vi "Delete Device Record.vi"(8 "error in (no error)":errorcluster, 10 "Device":string, 11 "Configuration in":refnum<class "Configuration.lvclass">) -> (0 "error out":errorcluster, 3 "Configuration out":refnum<class "Configuration.lvclass">)   [LabVIEW 2023, in "Configuration.lvlib" / "Configuration.lvclass"]
uses:
  Library/Configuration.lvclass
  Library/Configuration.lvclass/Configuration.ctl
  <vilib>/Utility/config.llb/NI_LVConfig.lvlib
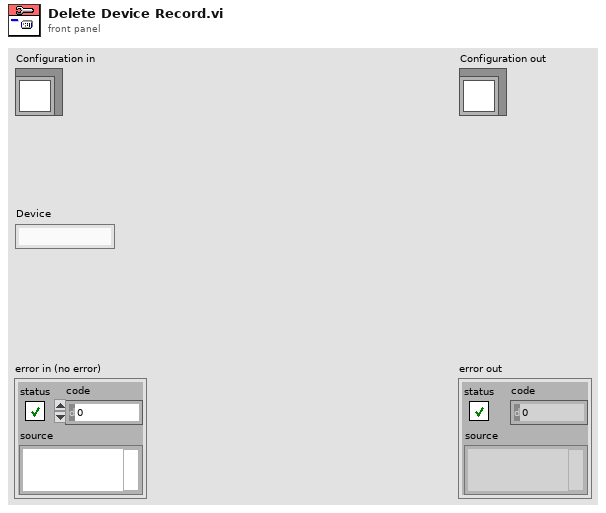
[diagram p1: front panel]
types:
  T1 = typedef "NI_LVConfig.lvlib/Config Data RefNum.ctl" = refnum<k1>
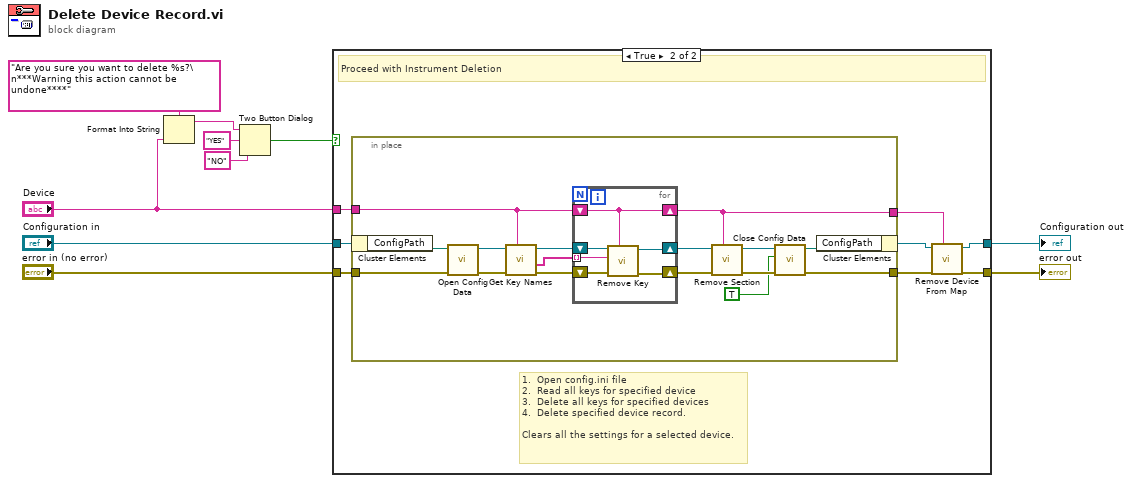
[diagram p0: block diagram]
diagram:
  n1 = Format Into String(format string="Are you sure you want to delete %s?\n***Warning this action cannot be undone****", "Device") -> (resulting string=w9:string)  [unwired: 2 in, 1 out]
  n2 = Two Button Dialog(message=w9, 1:"NO" ("F button name (\"Cancel\")"), 2:"YES" ("T button name (\"OK\")")) -> (T button?=w2:bool)
  n3 = case shown="True" w2 {
    tunnel: "Configuration in" -> [w12 w20]
    tunnel: [w12 w15] -> w5
    tunnel: "error in (no error)" -> [w11 w19]
    tunnel: [w11 w16] -> w4
    tunnel: "Device" -> [_ w18]
    frame False {
      # "Cancel Instrument deletion"
    }
    frame True {
      # "1.  Open config.ini file\n2.  Read all keys for specified device\n3.  Delete all keys for specified devices\n4.  Delete specified device record.\n\nClears all the settings for a selected device."
      # "Proceed with Instrument Deletion"
      n4 = in-place {
        in-place-border: w19 -> [w24]
        in-place-border: [w23] -> w17
        in-place-border: w18 -> [w22]
        in-place-border: [w21] -> w13
        n5 = in-place-cluster #1(w20) -> ("ConfigPath"=w36:path)
        n6 = call <vilib>:"Open Config Data.vi"("error in (no error)"=w24, "configuration file path"=w36) -> ("error out"=w35:errorcluster, "refnum"=w34:T1)  [unwired: 7 in, 1 out]
        n7 = call <vilib>:"Get Key Names.vi"("section"=w22, "error in (no error)"=w35, "refnum"=w34) -> ("error out"=w33:errorcluster, "key names"=w32:string[], "refnum out"=w31:T1)  [unwired: 5 in, 1 out]
        n8 = for {
          shift-right: [w41] -> w30
          shift-left: w33 -> [w42]
          tunnel: w32 -> [w40] mode=indexing
          shift-right: [w38] -> w29
          shift-left: w31 -> [w39]
          shift-right: [w37] -> w21
          shift-left: w22 -> [w37]
          # "Delete all settings"
          n9 = call <vilib>:"Remove Key.vi"("section"=w37, "error in (no error)"=w42, "key"=w40, "refnum"=w39) -> ("error out"=w41:errorcluster, "refnum out"=w38:T1)  [unwired: 5 in, 1 out]
        }
        n10 = call <vilib>:"Remove Section.vi"("section"=w21, "error in (no error)"=w30, "refnum"=w29) -> ("error out"=w28:errorcluster, "refnum out"=w27:T1)  [unwired: 6 in, 1 out]
        n11 = call <vilib>:"Close Config Data.vi"("error in (no error)"=w28, "write file if changed (T)"=TRUE, "refnum"=w27) -> ("error out"=w23:errorcluster, "file path"=w26:path)  [unwired: 7 in]
        n12 = in-place-cluster #1("ConfigPath"=w26) -> (w14:refnum<class "Configuration.lvclass">)
      }
      n13 = call "Remove Device From Map.vi"("Device"=w13, "error in (no error)"=w17, "Configuration in"=w14) -> ("error out"=w16:errorcluster, "Configuration out"=w15:refnum<class "Configuration.lvclass">)  [unwired: 7 in]
    }
  }
  "error out" <- w4
  "Configuration out" <- w5
